vi "SPI Flash Erase Sector.vi"(7 "NumSector":i32, 9 "StartSector":i32, 10 "SPIIndex":i32, 11 "DevHandle":i32) -> (3 "function return":i32)   [LabVIEW 2010, in "usb2spi.lvlib"]
doc: "int WINAPI SPI_FlashEraseSector(int DevHandle,int SPIIndex,int StartSector,int NumSector);"
uses:
  usb2spi.lvlib
  USB2XXX/trunk/USB2XXX/USB2XXX/vs2010/Release/USB2XXX.dll
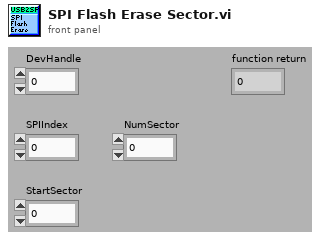
[diagram p1: front panel]
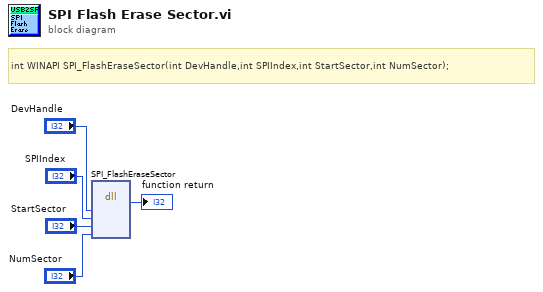
[diagram p0: block diagram]
diagram:
  # "int WINAPI SPI_FlashEraseSector(int DevHandle,int SPIIndex,int StartSector,int NumSector);"
  n1 = dll-call lib="E:/OtherWork/STM32/USB2XXX/trunk/USB2XXX/USB2XXX/vs2010/Release/USB2XXX.*" fn="SPI_FlashEraseSector"("DevHandle"="DevHandle", "SPIIndex"="SPIIndex", "StartSector"="StartSector", "NumSector"="NumSector") -> (→"function return":i32)  [unwired: 7 in, 2 out]
